vi "Save_Files_GCFS.vi"(3 "error in":errorcluster, 4 "Enum":enum16{"Freezing_Data", "Sample_Data"}(ring)=enum."Sample_Data", 5 "Array":string[][](array[string]), 6 "file path (use dialog)":path) -> (0 "error out":errorcluster, 2 "path":path)   [LabVIEW 2024]
uses:
  <vilib>/Utility/file.llb/Write Delimited Spreadsheet (string).vi
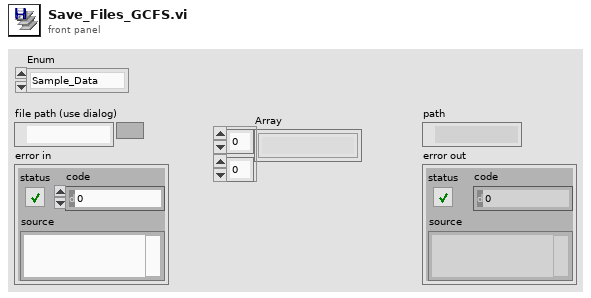
[diagram p1: front panel]
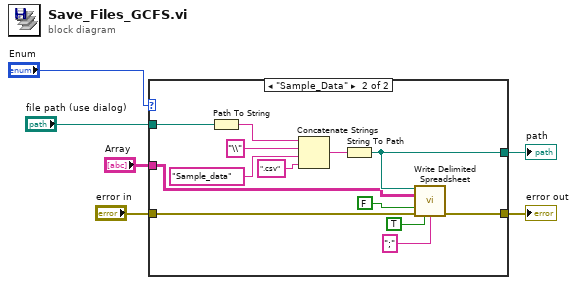
[diagram p0: block diagram]
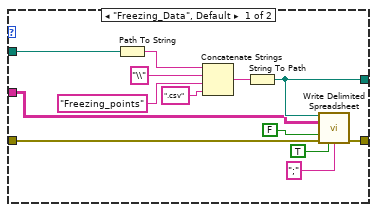
[diagram p2: hidden frame]
diagram:
  n1 = case shown="\"Sample_Data\"" "Enum" {
    tunnel: [w12 w30] -> w6
    tunnel: "error in" -> [w10 w29]
    tunnel: "file path (use dialog)" -> [w9 w23]
    tunnel: [w11 w22] -> w2
    tunnel: "Array" -> [w7 w20]
    frame "Freezing_Data", Default {
      n2 = Path To String(path=w9) -> (string=w14:string)
      n3 = Concatenate Strings(w14, "\\" ("string"), "Freezing_points" ("string"), ".csv" ("string")) -> (w17:string)
      n4 = String To Path(string=w17) -> (path=w11:path)
      n5 = call-poly <vilib>:"Write Delimited Spreadsheet.vi"("file path (dialog if empty)"=w11, "2D data"=w7, "append to file? (new file:F)"=FALSE, "error in (no error)"=w10, "transpose? (no:F)"=TRUE, "delimiter (\\t)"=";" ("delimiter (\\t)")) -> ("error out"=w12:errorcluster)  [unwired: 8 in, 1 out]
    }
    frame "Sample_Data" {
      n6 = Path To String(path=w23) -> (string=w24:string)
      n7 = Concatenate Strings(w24, "\\" ("string"), "Sample_data" ("string"), ".csv" ("string")) -> (w28:string)
      n8 = String To Path(string=w28) -> (path=w22:path)
      n9 = call-poly <vilib>:"Write Delimited Spreadsheet.vi"("file path (dialog if empty)"=w22, "2D data"=w20, "append to file? (new file:F)"=FALSE, "error in (no error)"=w29, "transpose? (no:F)"=TRUE, "delimiter (\\t)"=";" ("delimiter (\\t)")) -> ("error out"=w30:errorcluster)  [unwired: 8 in, 1 out]
    }
  }
  "path" <- w2
  "error out" <- w6
